vi "Try Match Abort.vi"(8 "error in":errorcluster, 10 "Data":u8[](array[numeric]), 11 "SDO Transfer in":refnum<class "SDO Transfer.lvclass">) -> (0 "error out":errorcluster, 2 "Success":bool, 3 "SDO Transfer out":refnum<class "SDO Transfer.lvclass">)   [LabVIEW 2020, in "CANopen.lvlib" / "SDO Manager.lvlib" / "SDO Transfer.lvclass"]
uses:
  SDO Transfer/SDO Transfer.lvclass
  SDO Transfer/SDO Transfer.lvclass/SDO Transfer.ctl
  SDO Transfer/SDO abort code.ctl
  Typedefs/SDO Result.ctl
  SDO Transfer/SDO Transfer Result.ctl
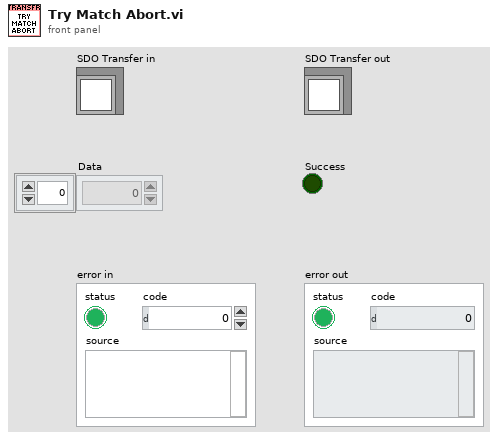
[diagram p1: front panel]
types:
  T1 = typedef "CANopen.lvlib/SDO Manager.lvlib/SDO Transfer.lvclass/SDO Transfer Result.ctl" = cluster{"SDO Result":T2, "Error":errorcluster}
  T2 = typedef "CANopen.lvlib/SDO Manager.lvlib/SDO Transfer.lvclass/SDO Result.ctl" = cluster{"Success":bool, "SDO abort code":cluster{"Null":bool, "Value":T3}, "Data":cluster{"Null":bool, "Data":u8[]}}
  T3 = typedef "CANopen.lvlib/SDO Manager.lvlib/SDO Transfer.lvclass/SDO abort code.ctl" = u32
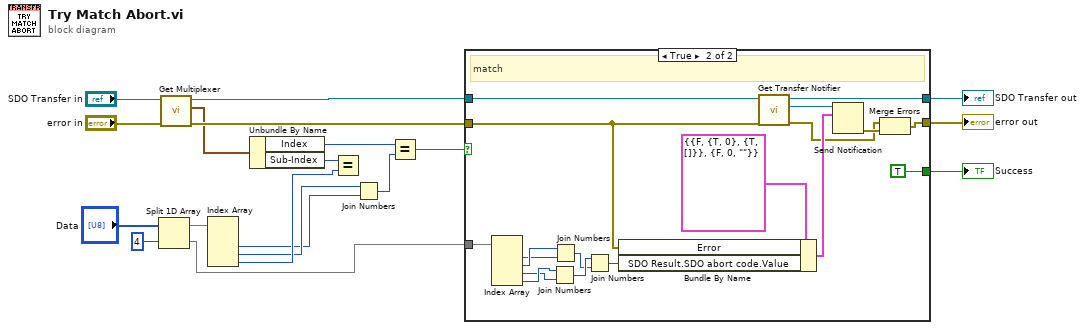
[diagram p0: block diagram]
diagram:
  n1 = Split 1D Array(array="Data", index=4) -> (first subarray=w6:u8[], second subarray=w4:u8[])
  n2 = call "Get Multiplexer.vi"("error in"="error in", "SDO Transfer in"="SDO Transfer in") -> ("error out"=w11:errorcluster, "Multiplexer"=w8:cluster{"Index":u16, "Sub-Index":u8}, "SDO Transfer out"=w9:refnum<class "SDO Transfer.lvclass">)  [unwired: 7 in]
  n3 = Index Array(array=w6) -> (element #2=w1:u8, element #3=w2:u8, element #4=w3:u8)  [unwired: 4 in, 1 out]
  n4 = Unbundle By Name(w8) -> ("Index"=w16:u16, "Sub-Index"=w17:u8)
  n5 = Equal?(x=w17, y=w3) -> ()  [unwired: 1 out]
  n6 = Join Numbers(hi=w2, lo=w1) -> ((hi.lo)=w18:u16)
  n7 = Equal?(x=w16, y=w18) -> (x = y?=w19:bool)
  n8 = case shown="True" w19 {
    tunnel: w11 -> [w21 w24]
    tunnel: w9 -> [w20 w37]
    tunnel: [w20 w35] -> w13
    tunnel: [w21 w23] -> w14
    tunnel: [_ TRUE] -> w15
    tunnel: w4 -> [_ w30]
    frame False {
      # "no match"
    }
    frame True {
      # "match"
      n9 = Index Array(array=w30) -> (element #1=w26:u8, element #2=w27:u8, element #3=w28:u8, element #4=w29:u8)  [unwired: 4 in]
      n10 = Join Numbers(hi=w29, lo=w28) -> ((hi.lo)=w39:u16)
      n11 = Join Numbers(hi=w27, lo=w26) -> ((hi.lo)=w38:u16)
      n12 = Join Numbers(hi=w39, lo=w38) -> ((hi.lo)=w33:u32)
      n13 = Bundle By Name(cluster=T1 {"SDO Result"={"Success"=FALSE, "SDO abort code"={"Null"=TRUE, "Value"=0}, "Data"={"Null"=TRUE, "Data"=[]}}, "Error"={"status"=FALSE, "code"=0, "source"=""}} ("SDO Transfer Result"), "Error"=w24, "SDO Result.SDO abort code.Value"=w33) -> (w34:T1)
      n14 = call "Get Transfer Notifier.vi"("error in"=w24, "SDO Transfer in"=w37) -> ("error out"=w22:errorcluster, "SDO Transfer Notifier"=w36:refnum<notifier>, "SDO Transfer out"=w35:refnum<class "SDO Transfer.lvclass">)  [unwired: 7 in]
      n15 = Send Notification(notification=w34, notifier=w36) -> (error out=w32:errorcluster)  [unwired: 1 in, 1 out]
      n16 = Merge Errors(w22, w32) -> (w23:errorcluster)
    }
  }
  "Success" <- w15
  "error out" <- w14
  "SDO Transfer out" <- w13
